vi "Pololu.Mgr - Send Message to Pololu.vi"(6 "Value":u16, 8 "error in (no error)":errorcluster, 9 "Channel":u8, 10 "Command":T1, 11 "PololuCtrl in":refnum<class "PololuCtrl.lvclass">) -> (0 "error out":errorcluster, 2 "Response":u16, 3 "PololuCtrl out":refnum<class "PololuCtrl.lvclass">)   [LabVIEW 2018, in "PololuCtrl.lvclass"]
uses:
  PololuCtrl.lvclass
  SubVIs/Pololu.Commands.ctl
  PololuCtrl.lvclass/PololuCtrl.ctl
  SubVIs/Pololu.Message Byte Defs.ctl
  Serial Port/Class/SerialPort.lvclass
panel:
  # "Position is quarter us\ni.e. for 1500us: 1500 X 4 = 6000\n\nSpeed is in 0.25us/10ms\nAccel is in  0.25us/10ms/80ms"
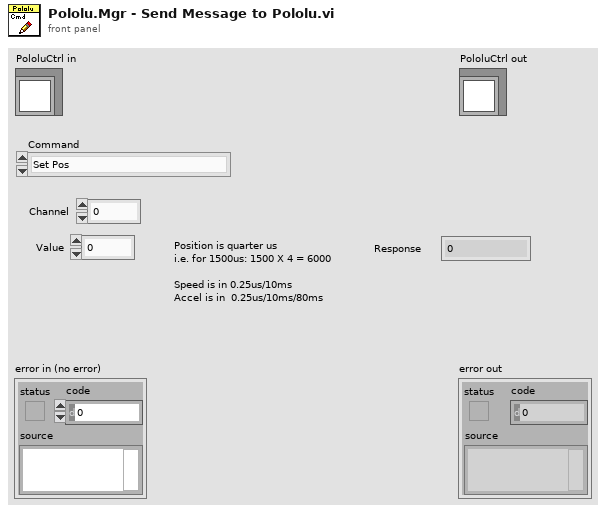
[diagram p1: front panel]
types:
  T1 = typedef "Pololu.Commands.ctl" = enum16{"Set Pos", "Set Speed", "Set Accel", "Get Pos", "Get Mov Status", "Get Errors"}
  T2 = cluster{"Command":T1, "Channel":u8, "Value":u16, "Response":u16, "Bytes":u8[], "Query":bool}
  T3 = typedef "Pololu.Message Byte Defs.ctl" = u8
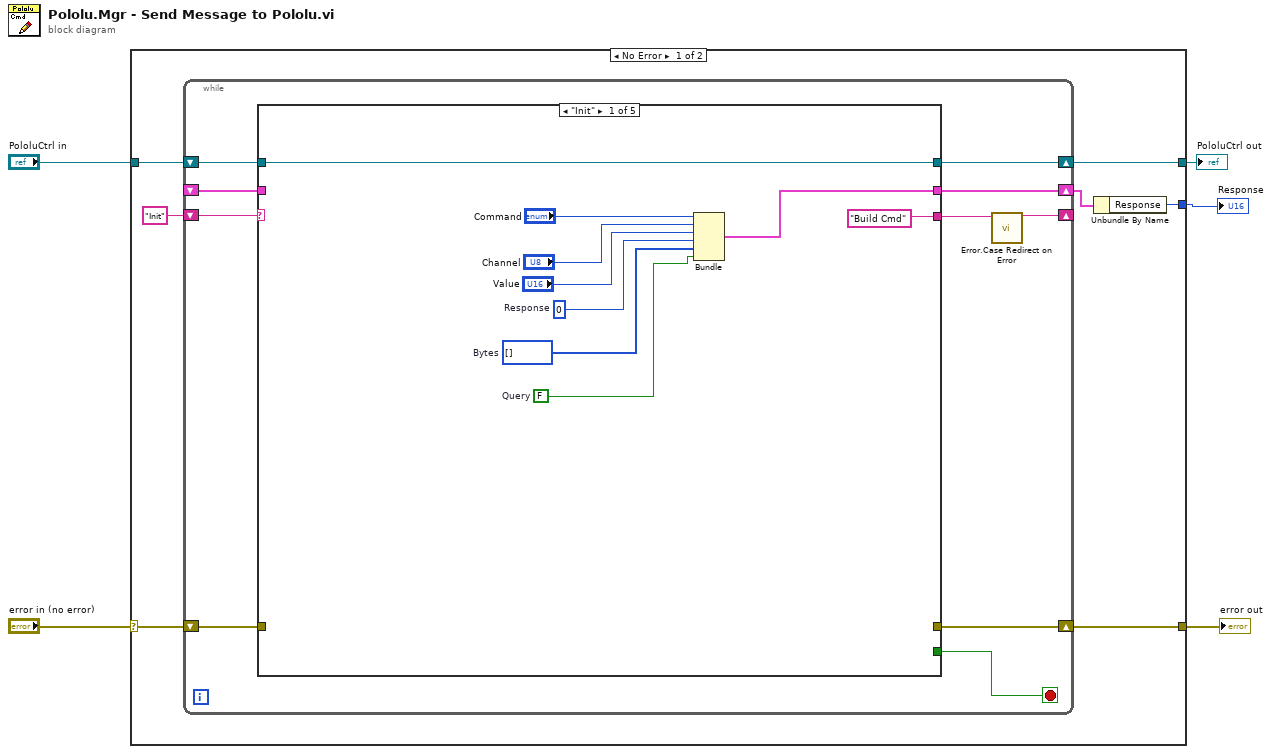
[diagram p0: block diagram]
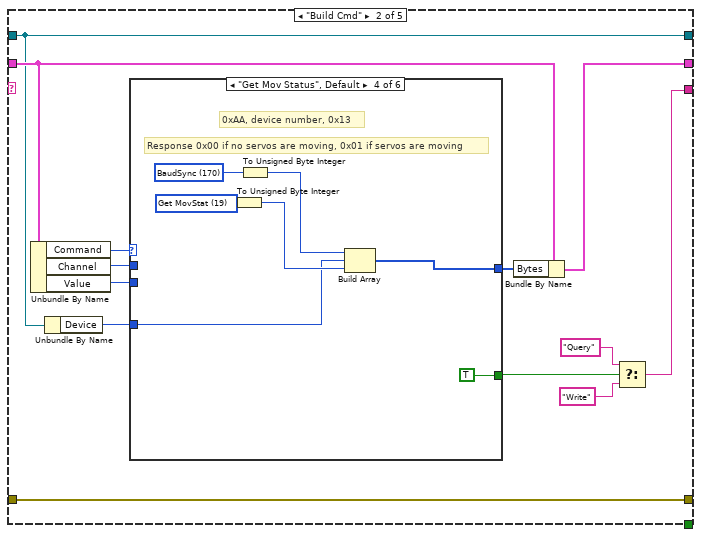
[diagram p2: hidden frame]
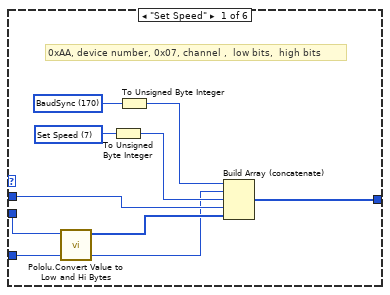
[diagram p3: hidden frame]
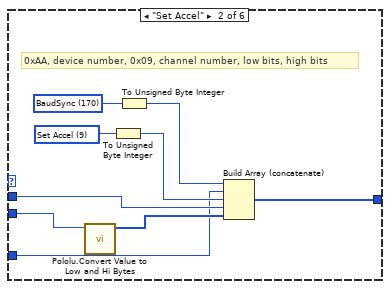
[diagram p4: hidden frame]
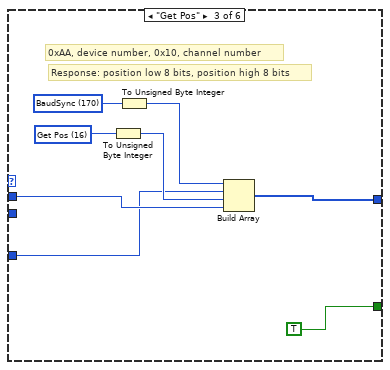
[diagram p5: hidden frame]
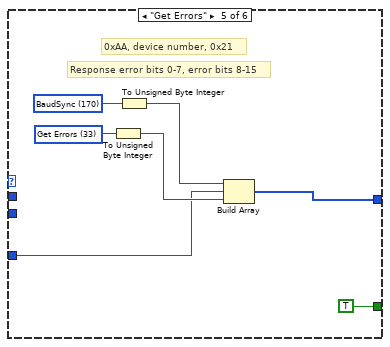
[diagram p6: hidden frame]
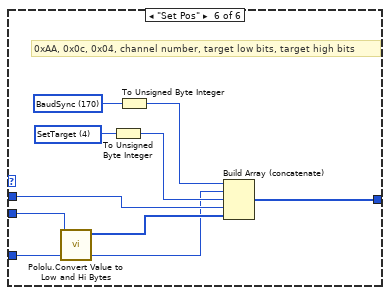
[diagram p7: hidden frame]
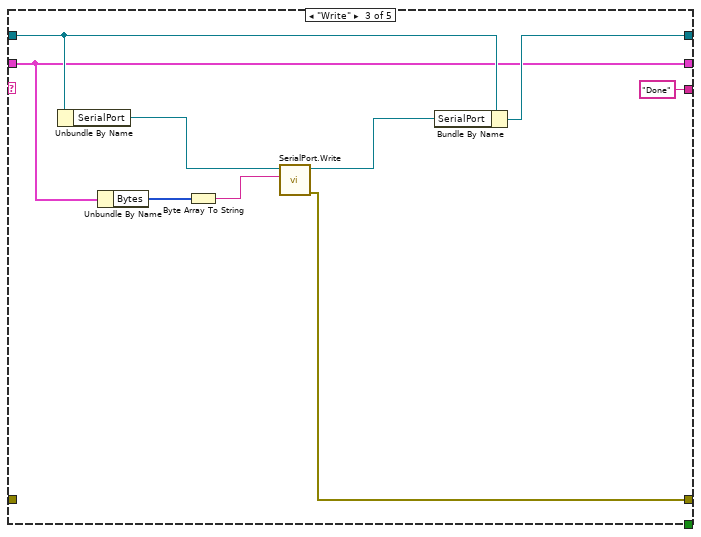
[diagram p8: hidden frame]
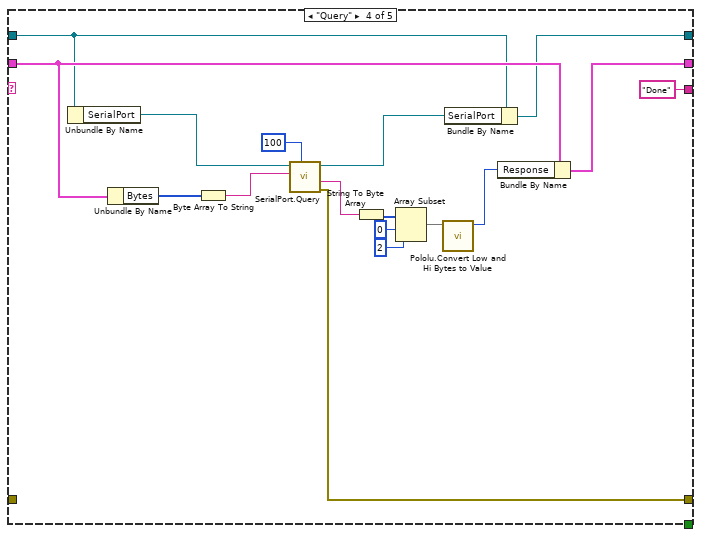
[diagram p9: hidden frame]
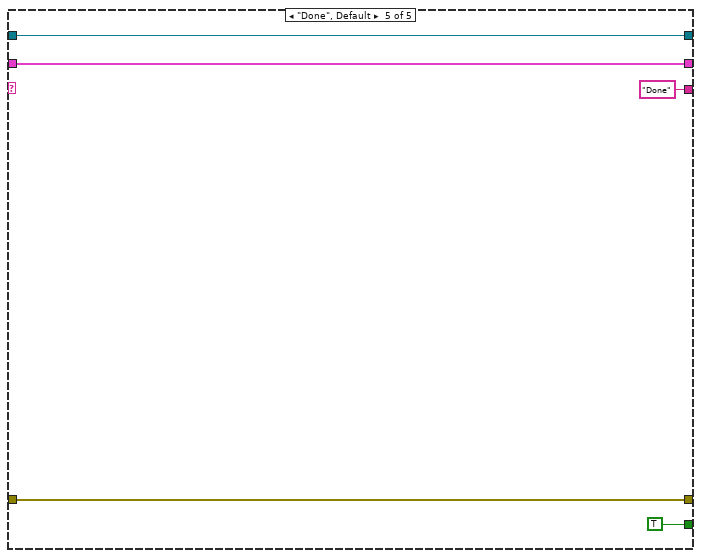
[diagram p10: hidden frame]
diagram:
  n1 = case shown="No Error" "error in (no error)" {
    selector: "error in (no error)" -> [w11 w126]
    tunnel: [w6 w126] -> w4
    tunnel: [w10 w125] -> w2
    tunnel: "PololuCtrl in" -> [w12 w125]
    tunnel: [w7 _] -> w1
    frame No Error {
      n2 = while {
        shift-right: [w21] -> w10
        shift-left: w12 -> [w22]
        shift-right: [w14] -> w6
        shift-left: w11 -> [w15]
        shift-right: [w18] -> _
        shift-left: "Init" -> [w19]
        shift-right: [w16] -> w8
        shift-left: _ -> [w20]
        stop <- w13 stop-if-true
        n3 = case shown="\"Init\"" w19 {
          tunnel: w22 -> [w31 w33 w99 w115 w124]
          tunnel: [w31 w33 w100 w116 w124] -> w21
          tunnel: w20 -> [_ w42 w95 w117 w121]
          tunnel: ["Build Cmd" w34 "Done" "Done" "Done"] -> w17
          tunnel: [w24 w43 w95 w118 w121] -> w16
          tunnel: w15 -> [_ w44 _ _ w122]
          tunnel: [_ w44 w96 w105 w122] -> w14
          tunnel: [_ _ _ _ TRUE] -> w13
          frame "Init" {
            w26 = u16 0  # Response
            w23 = FALSE  # Query
            w25 = u8[] []  # Bytes
            n4 = Bundle("Command"="Command", "Channel"="Channel", "Value"="Value", "Response"=w26, "Bytes"=w25, "Query"=w23) -> (w24:T2)  [unwired: 1 in]
          }
          frame "Build Cmd" {
            n5 = Unbundle By Name(w42) -> ("Command"=w41:T1, "Channel"=w40:u8, "Value"=w39:u16)
            n6 = Unbundle By Name(w33) -> ("Device"=w32:u8)
            n7 = case shown="\"Get Mov Status\", Default" w41 {
              tunnel: w40 -> [w50 w59 w67 _ _ w90]
              tunnel: w39 -> [w49 w58 _ _ _ w89]
              tunnel: [w51 w60 w68 w75 w82 w91] -> w38
              tunnel: [_ _ TRUE TRUE TRUE _] -> w37
              tunnel: w32 -> [w45 w54 w63 w71 w78 w85]
              frame "Set Speed" {
                w46 = T3 7 items=["BaudSync"=170, "SetTarget"=4, "Set Speed"=7, "Set Accel"=9, "Get Pos"=16, "Get MovStat"=19, "Get Errors"=33] ("Cmds")
                w47 = T3 170 items=["BaudSync"=170, "SetTarget"=4, "Set Speed"=7, "Set Accel"=9, "Get Pos"=16, "Get MovStat"=19, "Get Errors"=33] ("Cmds")
                # "0xAA, device number, 0x07, channel ,  low bits,  high bits"
                n8 = call "Pololu.Convert Value to Low and Hi Bytes.vi"("Value"=w49) -> ("Low_Hi Bytes"=w48:u8[])  [unwired: 10 in]
                n9 = To Unsigned Byte Integer(number=w46) -> (unsigned 8bit integer=w52:T3)
                n10 = To Unsigned Byte Integer(number=w47) -> (unsigned 8bit integer=w53:T3)
                n11 = Build Array (concatenate)(w53, w45, w52, w50, w48) -> (w51:T3[])
              }
              frame "Set Accel" {
                w55 = T3 9 items=["BaudSync"=170, "SetTarget"=4, "Set Speed"=7, "Set Accel"=9, "Get Pos"=16, "Get MovStat"=19, "Get Errors"=33] ("Cmds")
                w56 = T3 170 items=["BaudSync"=170, "SetTarget"=4, "Set Speed"=7, "Set Accel"=9, "Get Pos"=16, "Get MovStat"=19, "Get Errors"=33] ("Cmds")
                # "0xAA, device number, 0x09, channel number, low bits, high bits"
                n12 = call "Pololu.Convert Value to Low and Hi Bytes.vi"("Value"=w58) -> ("Low_Hi Bytes"=w57:u8[])  [unwired: 10 in]
                n13 = To Unsigned Byte Integer(number=w55) -> (unsigned 8bit integer=w61:T3)
                n14 = To Unsigned Byte Integer(number=w56) -> (unsigned 8bit integer=w62:T3)
                n15 = Build Array (concatenate)(w62, w54, w61, w59, w57) -> (w60:T3[])
              }
              frame "Get Pos" {
                w65 = T3 16 items=["BaudSync"=170, "SetTarget"=4, "Set Speed"=7, "Set Accel"=9, "Get Pos"=16, "Get MovStat"=19, "Get Errors"=33] ("Cmds")
                w66 = T3 170 items=["BaudSync"=170, "SetTarget"=4, "Set Speed"=7, "Set Accel"=9, "Get Pos"=16, "Get MovStat"=19, "Get Errors"=33] ("Cmds")
                # "Response: position low 8 bits, position high 8 bits"
                # "0xAA, device number, 0x10, channel number"
                n16 = To Unsigned Byte Integer(number=w65) -> (unsigned 8bit integer=w69:T3)
                n17 = To Unsigned Byte Integer(number=w66) -> (unsigned 8bit integer=w70:T3)
                n18 = Build Array(w70, w63, w69, w67) -> (w68:T3[])
              }
              frame "Get Mov Status", Default {
                w73 = T3 19 items=["BaudSync"=170, "SetTarget"=4, "Set Speed"=7, "Set Accel"=9, "Get Pos"=16, "Get MovStat"=19, "Get Errors"=33] ("Cmds")
                w74 = T3 170 items=["BaudSync"=170, "SetTarget"=4, "Set Speed"=7, "Set Accel"=9, "Get Pos"=16, "Get MovStat"=19, "Get Errors"=33] ("Cmds")
                # "Response 0x00 if no servos are moving, 0x01 if servos are moving"
                # "0xAA, device number, 0x13"
                n19 = To Unsigned Byte Integer(number=w73) -> (unsigned 8bit integer=w76:T3)
                n20 = To Unsigned Byte Integer(number=w74) -> (unsigned 8bit integer=w77:T3)
                n21 = Build Array(w77, w71, w76) -> (w75:T3[])
              }
              frame "Get Errors" {
                w80 = T3 33 items=["BaudSync"=170, "SetTarget"=4, "Set Speed"=7, "Set Accel"=9, "Get Pos"=16, "Get MovStat"=19, "Get Errors"=33] ("Cmds")
                w81 = T3 170 items=["BaudSync"=170, "SetTarget"=4, "Set Speed"=7, "Set Accel"=9, "Get Pos"=16, "Get MovStat"=19, "Get Errors"=33] ("Cmds")
                # "Response error bits 0-7, error bits 8-15"
                # "0xAA, device number, 0x21"
                n22 = To Unsigned Byte Integer(number=w80) -> (unsigned 8bit integer=w83:T3)
                n23 = To Unsigned Byte Integer(number=w81) -> (unsigned 8bit integer=w84:T3)
                n24 = Build Array(w84, w78, w83) -> (w82:T3[])
              }
              frame "Set Pos" {
                w86 = T3 4 items=["BaudSync"=170, "SetTarget"=4, "Set Speed"=7, "Set Accel"=9, "Get Pos"=16, "Get MovStat"=19, "Get Errors"=33] ("Cmds")
                w87 = T3 170 items=["BaudSync"=170, "SetTarget"=4, "Set Speed"=7, "Set Accel"=9, "Get Pos"=16, "Get MovStat"=19, "Get Errors"=33] ("Cmds")
                # "0xAA, 0x0c, 0x04, channel number, target low bits, target high bits"
                n25 = call "Pololu.Convert Value to Low and Hi Bytes.vi"("Value"=w89) -> ("Low_Hi Bytes"=w88:u8[])  [unwired: 10 in]
                n26 = To Unsigned Byte Integer(number=w86) -> (unsigned 8bit integer=w92:T3)
                n27 = To Unsigned Byte Integer(number=w87) -> (unsigned 8bit integer=w93:T3)
                n28 = Build Array (concatenate)(w93, w85, w92, w90, w88) -> (w91:T3[])
              }
            }
            n29 = Bundle By Name(cluster=w42, "Bytes"=w38) -> (w43:T2)
            n30 = Select(t="Query", s=w37, f="Write") -> (s? t:f=w34:string)
          }
          frame "Write" {
            n31 = Unbundle By Name(w99) -> ("SerialPort"=w98:refnum<class "SerialPort.lvclass">)
            n32 = Unbundle By Name(w95) -> ("Bytes"=w101:u8[])
            n33 = Byte Array To String(unsigned byte array=w101) -> (string=w94:string)
            n34 = call "SerialPort.Write.vi"("Data"=w94, "SerialPort in"=w98) -> ("error out"=w96:errorcluster, "SerialPort out"=w97:refnum<class "SerialPort.lvclass">)  [unwired: 6 in, 2 out]
            n35 = Bundle By Name(cluster=w99, "SerialPort"=w97) -> (w100:refnum<class "PololuCtrl.lvclass">)
          }
          frame "Query" {
            n36 = Unbundle By Name(w115) -> ("SerialPort"=w114:refnum<class "SerialPort.lvclass">)
            n37 = Unbundle By Name(w117) -> ("Bytes"=w104:u8[])
            n38 = Byte Array To String(unsigned byte array=w104) -> (string=w103:string)
            n39 = call "SerialPort.Query.vi"("TimeOut"=u32 100, "Cmd"=w103, "SerialPort in"=w114) -> ("error out"=w105:errorcluster, "Response"=w111:string, "SerialPort out"=w113:refnum<class "SerialPort.lvclass">)  [unwired: 4 in, 2 out]
            n40 = String To Byte Array(string=w111) -> (unsigned byte array=w110:u8[])
            n41 = Array Subset(array=w110, index=0, length=2) -> (w107:u8[])
            n42 = call "Pololu.Convert Low and Hi Bytes to Value.vi"("Low_Hi Bytes"=w107) -> ("Value"=w106:u16)  [unwired: 10 in]
            n43 = Bundle By Name(cluster=w115, "SerialPort"=w113) -> (w116:refnum<class "PololuCtrl.lvclass">)
            n44 = Bundle By Name(cluster=w117, "Response"=w106) -> (w118:T2)
          }
          frame "Done", Default {
          }
        }
        n45 = call "Error.Case Redirect on Error.vi"("Next Case"=w17) -> ("Next Case Out"=w18:string)  [unwired: 10 in]
      }
      n46 = Unbundle By Name(w8) -> ("Response"=w7:u16)
    }
    frame Error {
    }
  }
  "error out" <- w4
  "PololuCtrl out" <- w2
  "Response" <- w1
